vi "Close and Open Polygon.vi"(9 "type":u16(ring) items=["Closed", "Open"], 10 "Y In":dbl[](array[numeric]), 11 "X In":dbl[](array[numeric])) -> (2 "Y Out":dbl[](array[numeric]), 3 "X Out":dbl[](array[numeric]))   [LabVIEW 2020, in "NI_AAL_Geometry.lvlib"]
uses:
  <vilib>/Analysis/NI_AAL_Geometry.lvlib
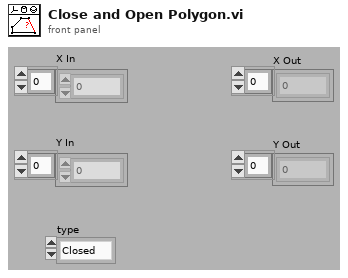
[diagram p1: front panel]
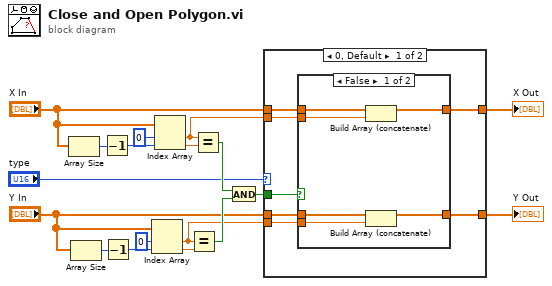
[diagram p0: block diagram]
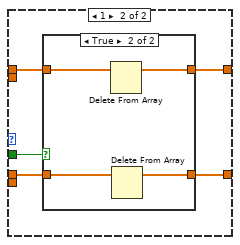
[diagram p3: hidden frame]
diagram:
  n1 = Array Size(array="X In") -> (size(s)=w18:i32)
  n2 = Array Size(array="Y In") -> (size(s)=w13:i32)
  n3 = Decrement(x=w18) -> (x-1=w1:i32)
  n4 = Decrement(x=w13) -> (x-1=w14:i32)
  n5 = Index Array(array="Y In", index #1=0 ("index"), index #2=w14) -> (element #1=w9:dbl, element #2=w12:dbl)
  n6 = Index Array(array="X In", index #1=0 ("index"), index #2=w1) -> (element #1=w8:dbl, element #2=w16:dbl)
  n7 = Equal?(x=w9, y=w12) -> (x = y?=w10:bool)
  n8 = Equal?(x=w8, y=w16) -> (x = y?=w11:bool)
  n9 = And(x=w11, y=w10) -> (x .and. y?=w7:bool)
  n10 = case shown="0, Default" "type" {
    tunnel: w9 -> [w22 _]
    tunnel: w8 -> [w24 _]
    tunnel: w7 -> [w19 w38]
    tunnel: "X In" -> [w25 w37]
    tunnel: "Y In" -> [w23 w36]
    tunnel: [w21 w35] -> w4
    tunnel: [w20 w34] -> w3
    frame 0, Default {
      n11 = case shown="False" w19 {
        tunnel: w25 -> [w27 w33]
        tunnel: [w30 w33] -> w21
        tunnel: w23 -> [w26 w32]
        tunnel: [w29 w32] -> w20
        tunnel: w24 -> [w31 _]
        tunnel: w22 -> [w28 _]
        frame False {
          n12 = Build Array (concatenate)(w27, w31) -> (w30:dbl[])
          n13 = Build Array (concatenate)(w26, w28) -> (w29:dbl[])
        }
        frame True {
        }
      }
    }
    frame 1 {
      n14 = case shown="True" w38 {
        tunnel: w37 -> [w40 w44]
        tunnel: w36 -> [w39 w43]
        tunnel: [w40 w42] -> w35
        tunnel: [w39 w41] -> w34
        frame False {
        }
        frame True {
          n15 = Delete From Array(array=w44) -> (array with subset deleted=w42:dbl[])  [unwired: 2 in, 1 out]
          n16 = Delete From Array(array=w43) -> (array with subset deleted=w41:dbl[])  [unwired: 2 in, 1 out]
        }
      }
    }
  }
  "X Out" <- w4
  "Y Out" <- w3
